vi "LastGameViewer.vi"(11 "GameData":T1) -> ()   [LabVIEW 2024]
uses:
  Controls/GameInfo.ctl
  Controls/E_Phases.ctl
panel:
  out "output array":string[][](array[string])
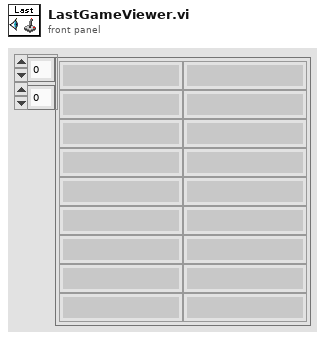
[diagram p1: front panel]
types:
  T1 = typedef "GameInfo.ctl" = cluster{"Player":string, "Opponent":string, "PArmy":string, "OArmy":string, "CP":dbl, "VP":dbl, "GameStart":timestamp, "GameEnd":timestamp, "BattleRound":dbl, "PrimaryMissionPoints":dbl, "SecondaryMissionPoints":dbl, "BattlePhase":T2, "Win":dbl, "Lose":dbl}
  T2 = typedef "E_Phases.ctl" = enum16{"Null/Error", "Command Phase", "Movement Phase", "Shooting Phase", "Charge Phase", "Fight Phase", "Secondary Scoring", "Enemy Command Phase", "Enemy Movement Phase", "Enemy Shooting Phase", "Enemy Charge Phase", "Enemy Fight Phase", "Enemy Secondary Scoring"}
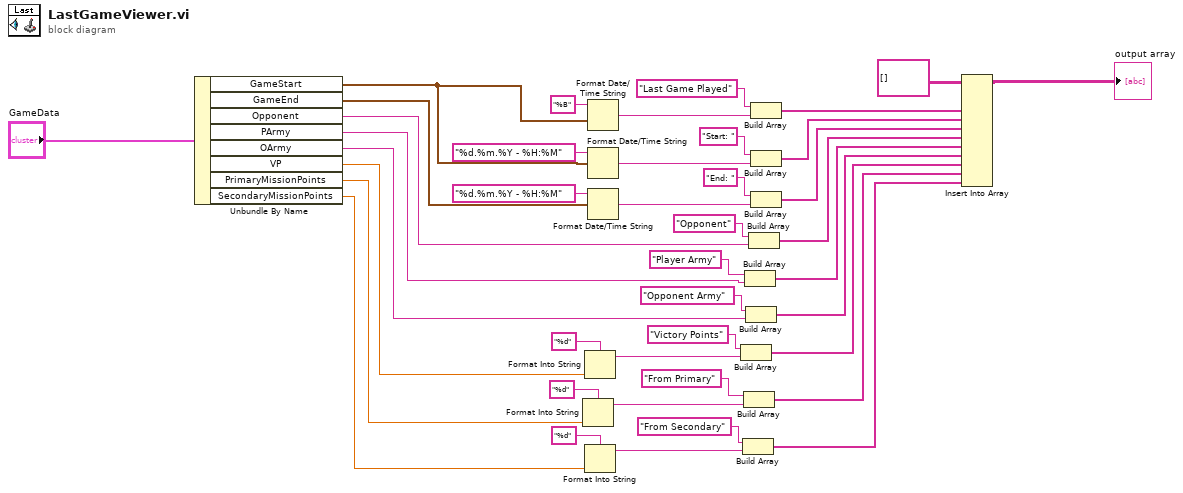
[diagram p0: block diagram]
diagram:
  n1 = Unbundle By Name("GameData") -> ("GameStart"=w23:timestamp, "GameEnd"=w24:timestamp, "Opponent"=w25:string, "PArmy"=w26:string, "OArmy"=w27:string, "VP"=w28:dbl, "PrimaryMissionPoints"=w29:dbl, "SecondaryMissionPoints"=w30:dbl)
  n2 = Format Into String(format string="%d", w29) -> (resulting string=w3:string)  [unwired: 2 in, 1 out]
  n3 = Format Into String(format string="%d", w28) -> (resulting string=w2:string)  [unwired: 2 in, 1 out]
  n4 = Format Into String(format string="%d", w30) -> (resulting string=w4:string)  [unwired: 2 in, 1 out]
  n5 = Format Date/Time String(time format string (%c)="%B", seconds (now)=w23) -> (date/time string=w7:string)  [unwired: 1 in]
  n6 = Format Date/Time String(time format string (%c)="%d.%m.%Y - %H:%M", seconds (now)=w23) -> (date/time string=w6:string)  [unwired: 1 in]
  n7 = Format Date/Time String(time format string (%c)="%d.%m.%Y - %H:%M", seconds (now)=w24) -> (date/time string=w5:string)  [unwired: 1 in]
  n8 = Build Array("Victory Points" ("element"), w2) -> (w38:string[])
  n9 = Build Array("From Secondary" ("element"), w4) -> (w40:string[])
  n10 = Build Array("From Primary" ("element"), w3) -> (w39:string[])
  n11 = Build Array("Player Army" ("element"), w26) -> (w36:string[])
  n12 = Build Array("Opponent Army" ("element"), w27) -> (w37:string[])
  n13 = Build Array("Opponent" ("element"), w25) -> (w35:string[])
  n14 = Build Array("Last Game Played" ("element"), w7) -> (w32:string[])
  n15 = Build Array("Start: " ("element"), w6) -> (w33:string[])
  n16 = Build Array("End: " ("element"), w5) -> (w34:string[])
  n17 = Insert Into Array(array=string[][] [], new element #1=w32, new element #2=w33, new element #3=w34, new element #4=w35, new element #5=w36, new element #6=w37, new element #7=w38, new element #8=w39, new element #9=w40) -> (→"output array":string[][])  [unwired: 2 in]
